vi "Select stimulus.vi"(10 "Output freq (Hz)":dbl=50.0) -> (1 "cancelled":bool, 2 "output":dbl[][](array[numeric]), 3 "Stimulus":T1={"type"=enum."Zero", "sinfreq start"=0.0, "sinfreq end"=0.0, "sinamp start"=0.0, "sinamp end"=0.0, "noise freq lo"=0.0, "noise freq hi"=0.0, "noiseamp start"=0.0, "noiseamp end"=0.0, "stimdur"=100.0, "before dur"=20.0, "after dur"=30.0} {"noise freq hi" min=0.0 step=0.5; "noise freq lo" min=0.0 step=0.5; "noiseamp end" min=0.0 step=0.5; "noiseamp start" min=0.0 step=0.5})   [LabVIEW 2012]
uses:
  <vilib>/Analysis/NI_AALBase.lvlib
  Stimulus type.ctl
  Stimulus.ctl
  <vilib>/Analysis/1siggen.llb/Ramp Pattern by Samples.vi
panel:
  out "Waveform Graph":waveform(dbl)[](graph)=[{"t0"=timestamp(0 s since 1904-01-01), "dt"=inf, "Y"=[]}, {"t0"=timestamp(0 s since 1904-01-01), "dt"=inf, "Y"=[]}, {"t0"=timestamp(0 s since 1904-01-01), "dt"=inf, "Y"=[]}]
  in  "Cancel":bool
  in  "OK":bool
  in  "stim dur unit":enum16{"cycles", "sec"}(ring)
  in  "after":dbl[unit]=30.0 caption="After"
  in  "before":dbl[unit]=20.0 caption="Before"
  in  "stimdur":dbl=100.0 caption="Stimulus"
  in  "Stimulus type":T3(tab)=enum."Frequency sweep"
  in  "noisehifreq":dbl[unit]=10.0 caption="High cutoff"
  in  "noiseamp":dbl[unit] caption="Amplitude"
  in  "noiselofreq":dbl[unit] caption="Low cutoff"
  in  "sinamp":dbl[unit]=0.3490658503988659 caption="Amplitude"
  in  "sinfreq":dbl[unit]=1.0 caption="Frequency"
  in  "Hi freq cutoff":dbl[unit]=10.0 min=0.0 step=0.5
  in  "Lo freq cutoff":dbl[unit] min=0.0 step=0.5
  in  "Start noise":dbl[unit] caption="Start" min=0.0 step=0.008726646259971648
  in  "Frequency":dbl[unit]=1.0 min=0.0 step=0.05
  in  "Start amp":dbl[unit]=0.5235987755982988 caption="Start" min=0.0 step=0.017453292519943295
  in  "End amplitude":dbl[unit]=0.5235987755982988 caption="End" min=0.0 step=0.017453292519943295
  in  "End noise":dbl[unit] caption="End" min=0.0 step=0.008726646259971648
  in  "hi cutoff":dbl[unit]=10.0 caption="High cutoff"
  in  "noiseamp":dbl[unit] caption="Amplitude"
  in  "lo cutoff":dbl[unit] caption="Low cutoff"
  in  "endfreq":dbl[unit]=2.0 caption="End" min=0.0 step=0.05
  in  "startfreq":dbl[unit]=0.5 caption="Start" min=0.0 step=0.05
  in  "sinamp":dbl=30.0 caption="Amplitude" min=0.0 step=1.0
  # "Duration:"
  # "Just record baseline bursting with no stimulus"
  # "s"
  # "Signal:"
  # "Noise:"
  # "Signal:"
  # "Amplitude:"
  # "Noise:"
  # "Amplitude:"
  # "Signal:"
  # "Frequency:"
  # "Noise:"
  # "s"
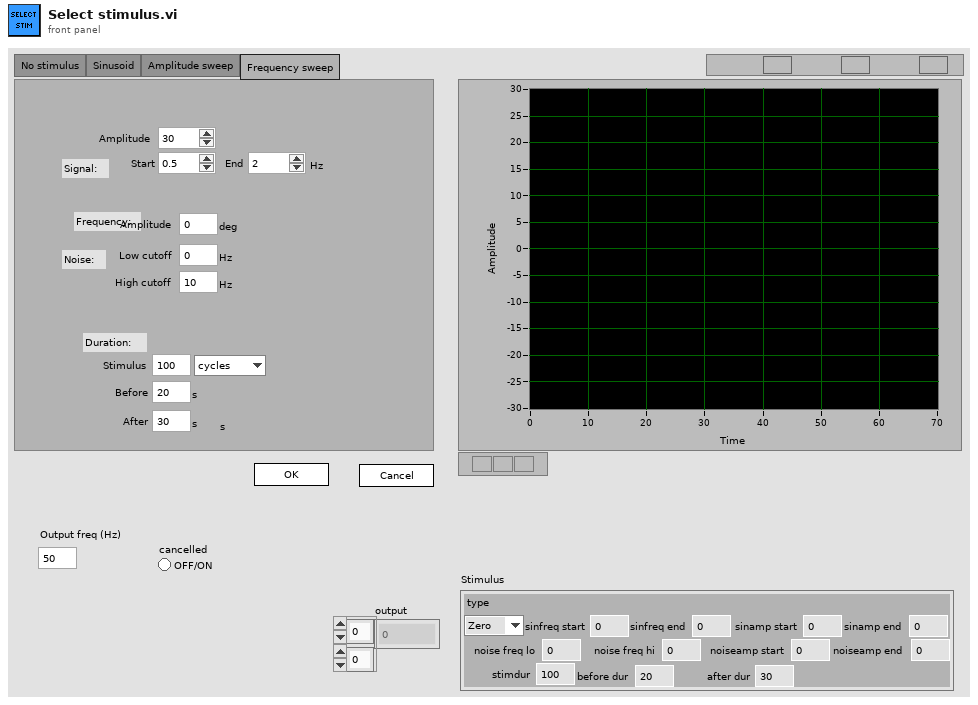
[diagram p1: front panel]
types:
  T1 = typedef "Stimulus.ctl" = cluster{"type":T2, "sinfreq start":dbl, "sinfreq end":dbl, "sinamp start":dbl, "sinamp end":dbl, "noise freq lo":dbl, "noise freq hi":dbl, "noiseamp start":dbl, "noiseamp end":dbl, "stimdur":dbl, "before dur":dbl, "after dur":dbl}
  T2 = typedef "Stimulus type.ctl" = enum16{"Zero", "Sine", "Frequency sweep", "Two frequency", "Amplitude sweep"}
  T3 = enum32{"No stimulus", "Sinusoid", "Amplitude sweep", "Frequency sweep"}
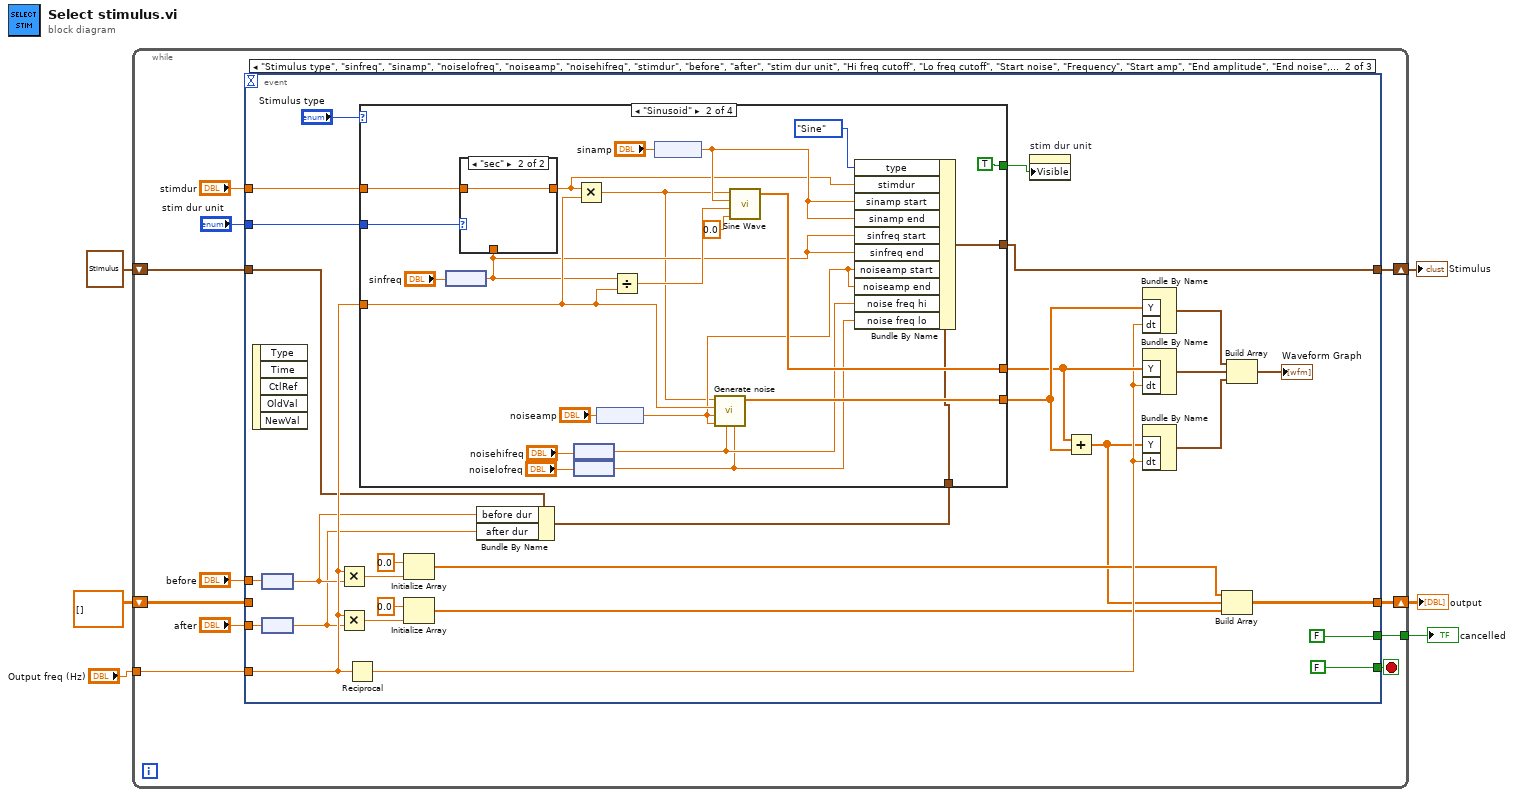
[diagram p0: block diagram]
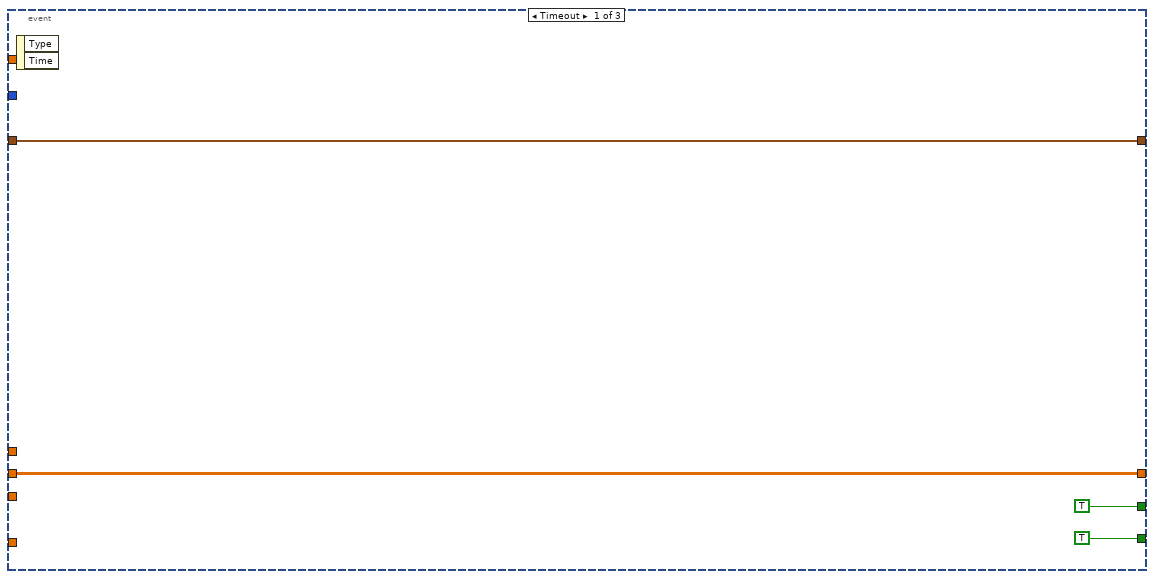
[diagram p2: hidden frame]
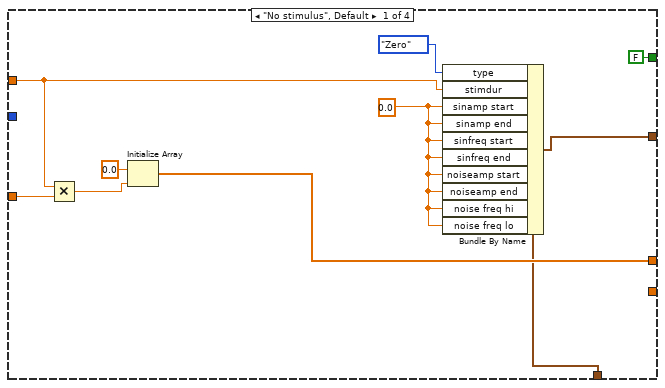
[diagram p3: hidden frame]
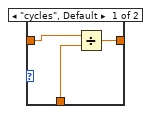
[diagram p4: hidden frame]
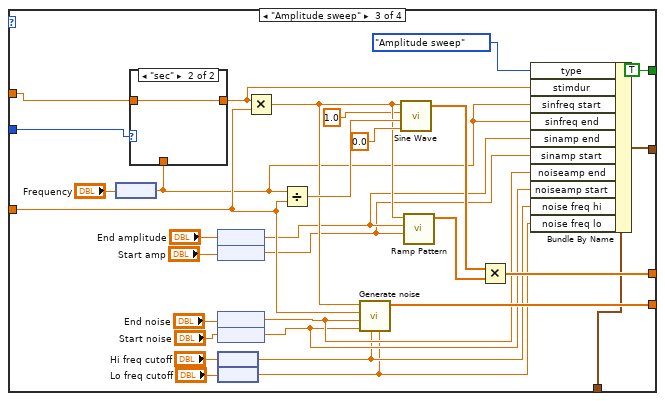
[diagram p5: hidden frame]
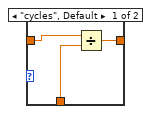
[diagram p6: hidden frame]
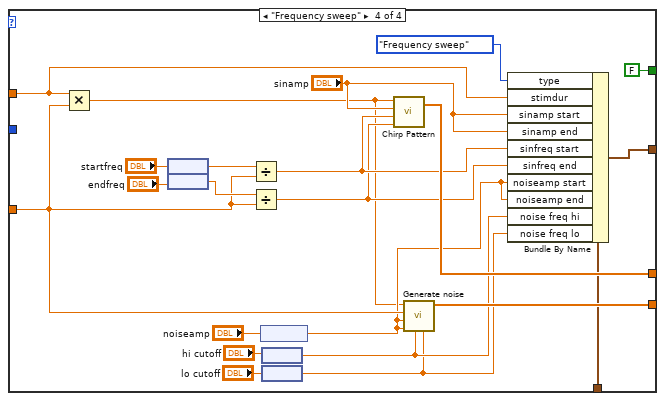
[diagram p7: hidden frame]
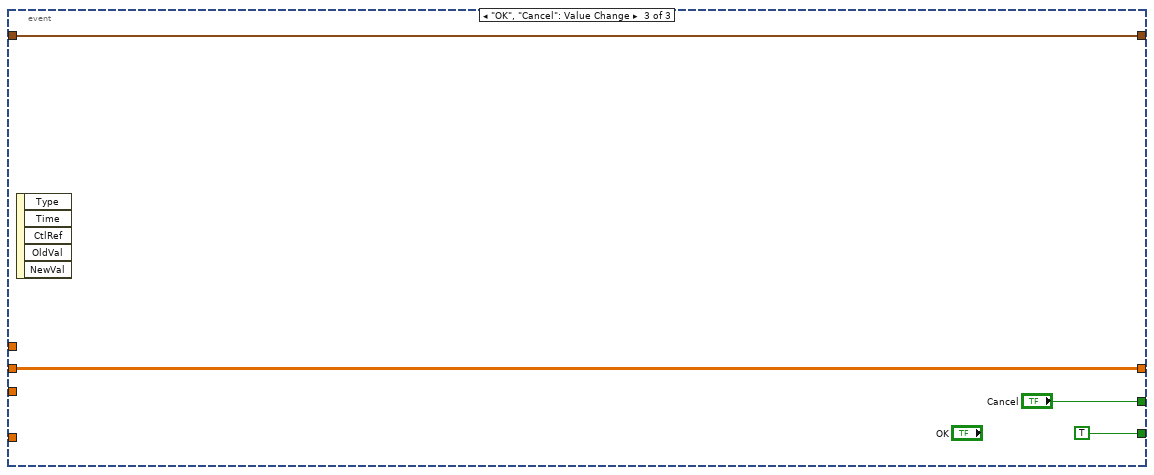
[diagram p8: hidden frame]
diagram:
  n1 = while {
    tunnel: "Output freq (Hz)" -> [w14]
    tunnel: [w12] -> w5
    shift-right: [w10] -> w4
    shift-left: T1 {"type"=enum."Zero", "sinfreq start"=0.0, "sinfreq end"=0.0, "sinamp start"=0.0, "sinamp end"=0.0, "noise freq lo"=0.0, "noise freq hi"=0.0, "noiseamp start"=0.0, "noiseamp end"=0.0, "stimdur"=0.0, "before dur"=0.0, "after dur"=0.0} ("Stimulus 2") -> [w7]
    shift-right: [w9] -> w1
    shift-left: dbl[][] [] -> [w8]
    stop <- w11 stop-if-true
    n2 = event shown="[1] \"Stimulus type\", \"sinfreq\", \"sinamp\", \"noiselofreq\", \"noiseamp\", \"noisehifreq\", \"stimdur\", \"before\", \"after\", \"stim dur unit\", \"Hi freq cutoff\", \"Lo freq cutoff\", \"Start noise\", \"Frequency\", \"Start amp\", \"End amplitude\", \"End noise\", \"sinamp\", \"startfreq\", \"endfreq\", \"lo cutoff\", \"noiseamp\", \"hi cutoff\": Value Change" {
      selector: _ -> [_ _ _]
      dyn-events: _ -> [_ _ _]
      timeout: _ -> [_ _ _]
      tunnel: "stimdur" -> [_ w49 _]
      tunnel: "before" -> [_ w48 _]
      tunnel: "after" -> [_ w47 _]
      tunnel: w14 -> [_ w42 _]
      tunnel: "stim dur unit" -> [_ w41 _]
      tunnel: [TRUE ("OK") FALSE ("OK") "Cancel"] -> w12
      tunnel: [TRUE ("OK") FALSE ("OK") TRUE ("OK")] -> w11
      tunnel: [w19 w36 w145] -> w10
      tunnel: [w18 w26 w144] -> w9
      tunnel: w8 -> [w18 _ w144]
      tunnel: w7 -> [w19 w22 w145]
      event Timeout {
        n3 = event-data() -> ()  [unwired: 1 in, 2 out]
      }
      event "Stimulus type", "sinfreq", "sinamp", "noiselofreq", "noiseamp", "noisehifreq", "stimdur", "before", "after", "stim dur unit", "Hi freq cutoff", "Lo freq cutoff", "Start noise", "Frequency", "Start amp", "End amplitude", "End noise", "sinamp", "startfreq", "endfreq", "lo cutoff", "noiseamp", "hi cutoff": Value Change {
        n4 = event-data() -> ()  [unwired: 1 in, 5 out]
        n5 = node(w48) -> (w25:dbl)
        n6 = node(w47) -> (w24:dbl)
        n7 = Multiply(x=w42, y=w25) -> (x*y=w45:dbl)
        n8 = Multiply(x=w42, y=w24) -> (x*y=w43:dbl)
        n9 = Reciprocal(x=w42) -> (1/x=w31:dbl)
        n10 = Initialize Array(0.0 ("element"), w45) -> (w29:dbl[])
        n11 = Initialize Array(0.0 ("element"), w43) -> (w28:dbl[])
        n12 = Bundle By Name(cluster=w22, "before dur"=w25, "after dur"=w24) -> (w23:T1)
        n13 = case shown="\"Sinusoid\"" "Stimulus type" {
          tunnel: w49 -> [w54 w82 w114 w122]
          tunnel: w42 -> [w59 w74 w111 w133]
          tunnel: [w57 w77 w104 w136] -> w33
          tunnel: w41 -> [_ w83 w102 _]
          tunnel: [FALSE ("Visible") TRUE ("Visible") TRUE ("Visible") FALSE ("Visible")] -> w38
          tunnel: [_ w71 w103 w135] -> w34
          tunnel: [w52 w63 w91 w126] -> w36
          tunnel: w23 -> [w51 w62 w90 w124]
          frame "No stimulus", Default {
            w53 = 0.0 ("sinamp start")
            n14 = Multiply(x=w54, y=w59) -> (x*y=w58:dbl)
            n15 = Initialize Array(0.0 ("element"), w58) -> (w57:dbl[])
            n16 = Bundle By Name(cluster=w51, "type"=Stimulus_type."Zero", "stimdur"=w54, "sinamp start"=w53, "sinamp end"=w53, "sinfreq start"=w53, "sinfreq end"=w53, "noiseamp start"=w53, "noiseamp end"=w53, "noise freq hi"=w53, "noise freq lo"=w53) -> (w52:T1)
          }
          frame "Sinusoid" {
            n17 = node("sinfreq") -> (w69:dbl)
            n18 = case shown="\"sec\"" w83 {
              tunnel: w82 -> [w85 w87]
              tunnel: [w86 w87] -> w61
              tunnel: w69 -> [w84 _]
              frame "cycles", Default {
                n19 = Divide(x=w85, y=w84) -> (x/y=w86:dbl)
              }
              frame "sec" {
              }
            }
            n20 = node("noisehifreq") -> (w66:dbl)
            n21 = node("noiselofreq") -> (w65:dbl)
            n22 = Multiply(x=w61, y=w74) -> (x*y=w64:dbl)
            n23 = node("noiseamp") -> (w67:dbl)
            n24 = Divide(x=w69, y=w74) -> (x/y=w79:dbl)
            n25 = node("sinamp") -> (w68:dbl)
            n26 = call "Generate noise.vi"("noisehifreq"=w65, "noiselofreq"=w66, 8:w67, "noise std"=w67, "input dt"=w74, "samples"=w64) -> ("noise"=w71:dbl[])  [unwired: 4 in, 1 out]
            n27 = call <vilib>:"Sine Wave.vi"("samples"=w64, "amplitude"=w68, "frequency"=w79, "phase in"=0.0) -> ("sine wave"=w77:dbl[])  [unwired: 1 in, 2 out]
            n28 = Bundle By Name(cluster=w62, "type"=Stimulus_type."Sine", "stimdur"=w61, "sinamp start"=w68, "sinamp end"=w68, "sinfreq start"=w69, "sinfreq end"=w69, "noiseamp start"=w67, "noiseamp end"=w67, "noise freq hi"=w66, "noise freq lo"=w65) -> (w63:T1)
          }
          frame "Amplitude sweep" {
            n29 = node("Frequency") -> (w98:dbl)
            n30 = case shown="\"sec\"" w102 {
              tunnel: w114 -> [w119 w121]
              tunnel: [w120 w121] -> w88
              tunnel: w98 -> [w118 _]
              frame "cycles", Default {
                n31 = Divide(x=w119, y=w118) -> (x/y=w120:dbl)
              }
              frame "sec" {
              }
            }
            n32 = node("End amplitude") -> (w97:dbl)
            n33 = node("Start amp") -> (w96:dbl)
            n34 = node("End noise") -> (w95:dbl)
            n35 = node("Start noise") -> (w94:dbl)
            n36 = node("Hi freq cutoff") -> (w93:dbl)
            n37 = node("Lo freq cutoff") -> (w92:dbl)
            n38 = Multiply(x=w88, y=w111) -> (x*y=w99:dbl)
            n39 = Divide(x=w98, y=w111) -> (x/y=w117:dbl)
            n40 = call "Generate noise.vi"("noisehifreq"=w92, "noiselofreq"=w93, 8:w94, "noise std"=w95, "input dt"=w111, "samples"=w99) -> ("noise"=w103:dbl[])  [unwired: 4 in, 1 out]
            n41 = call <vilib>:"Sine Wave.vi"("samples"=w99, "amplitude"=1.0, "frequency"=w117, "phase in"=0.0) -> ("sine wave"=w106:dbl[])  [unwired: 1 in, 2 out]
            n42 = call-poly <vilib>:"Ramp Pattern.vi"("start"=w96, "end"=w97, "samples"=w99) -> ("Ramp Pattern"=w105:dbl[])  [unwired: 7 in, 1 out]
            n43 = Multiply(x=w106, y=w105) -> (x*y=w104:dbl[])
            n44 = Bundle By Name(cluster=w90, "type"=Stimulus_type."Amplitude sweep", "stimdur"=w88, "sinfreq start"=w98, "sinfreq end"=w98, "sinamp end"=w97, "sinamp start"=w96, "noiseamp end"=w95, "noiseamp start"=w94, "noise freq hi"=w93, "noise freq lo"=w92) -> (w91:T1)
          }
          frame "Frequency sweep" {
            n45 = Multiply(x=w122, y=w133) -> (x*y=w123:dbl)
            n46 = node("startfreq") -> (w140:dbl)
            n47 = node("endfreq") -> (w134:dbl)
            n48 = Divide(x=w140, y=w133) -> (x/y=w130:dbl)
            n49 = Divide(x=w134, y=w133) -> (x/y=w129:dbl)
            n50 = node("noiseamp") -> (w125:dbl)
            n51 = node("hi cutoff") -> (w128:dbl)
            n52 = node("lo cutoff") -> (w127:dbl)
            n53 = call <vilib>:"Chirp Pattern.vi"("f2"=w129, "f1"=w130, "amplitude"="sinamp", "samples"=w123) -> ("Chirp Pattern"=w136:dbl[])  [unwired: 1 out]
            n54 = call "Generate noise.vi"("noisehifreq"=w127, "noiselofreq"=w128, 8:w125, "noise std"=w125, "input dt"=w133, "samples"=w123) -> ("noise"=w135:dbl[])  [unwired: 4 in, 1 out]
            n55 = Bundle By Name(cluster=w124, "type"=Stimulus_type."Frequency sweep", "stimdur"=w122, "sinamp start"="sinamp", "sinamp end"="sinamp", "sinfreq start"=w130, "sinfreq end"=w129, "noiseamp start"=w125, "noiseamp end"=w125, "noise freq hi"=w128, "noise freq lo"=w127) -> (w126:T1)
          }
        }
        n56 = property on="stim dur unit" class="Enum (strict)"("Visible"=w38) -> ()  [unwired: 2 in, 2 out]
        n57 = Add(x=w33, y=w34) -> (x+y=w27:dbl[])
        n58 = Bundle By Name("Y"=w34, "dt"=w31) -> (w35:waveform(dbl))  [unwired: 1 in]
        n59 = Bundle By Name("Y"=w33, "dt"=w31) -> (w32:waveform(dbl))  [unwired: 1 in]
        n60 = Bundle By Name("Y"=w27, "dt"=w31) -> (w30:waveform(dbl))  [unwired: 1 in]
        n61 = Build Array(w29, w27, w28) -> (w26:dbl[][])
        n62 = Build Array(w35, w32, w30) -> (→"Waveform Graph":waveform(dbl)[])
      }
      event "OK", "Cancel": Value Change {
        n63 = event-data() -> ()  [unwired: 1 in, 5 out]
      }
    }
  }
  "cancelled" <- w5
  "Stimulus" <- w4
  "output" <- w1
